vi "createItemsInstances.vi"(8 "error in (no error)":errorcluster, 11 "reference in":refnum<class "Items Controller.lvclass">) -> (0 "error out":errorcluster, 3 "reference out":refnum<class "Items Controller.lvclass">)   [LabVIEW 2016, in "Items Controller.lvclass"]
uses:
  Items Controller.lvclass
  storageSheets.ctl
  APP/item_class/item.lvclass
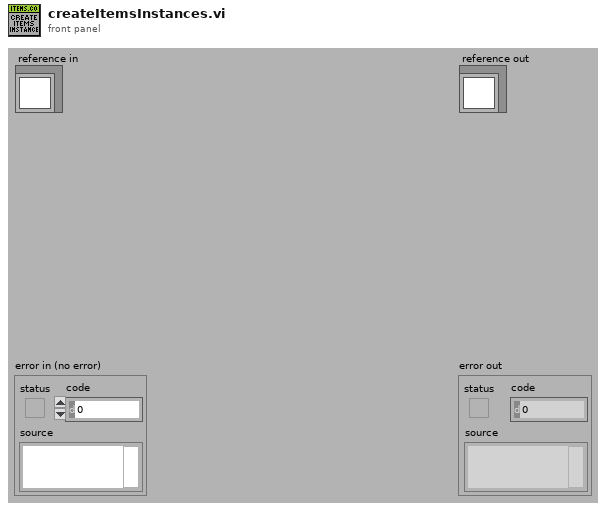
[diagram p1: front panel]
types:
  T1 = typedef "Items Controller.lvclass/storageSheets.ctl" = enum16{"check-in", "check-out", "storage"}
  T2 = typedef "Items Controller.lvclass/ObjectAttributesRef.ctl" = refnum<data-value>
  T3 = typedef "Items Controller.lvclass/ObjectAttributes.ctl" = cluster{"MyAttribute":dbl, "data":string[][][], "file_controller_ref":refnum<class "File Controller.lvclass">, "checkIN_ref":refnum<class "checkIN.lvclass">, "checkOUT_ref":refnum<class "checkOUT.lvclass">, "item_ref":refnum<class "item.lvclass">}
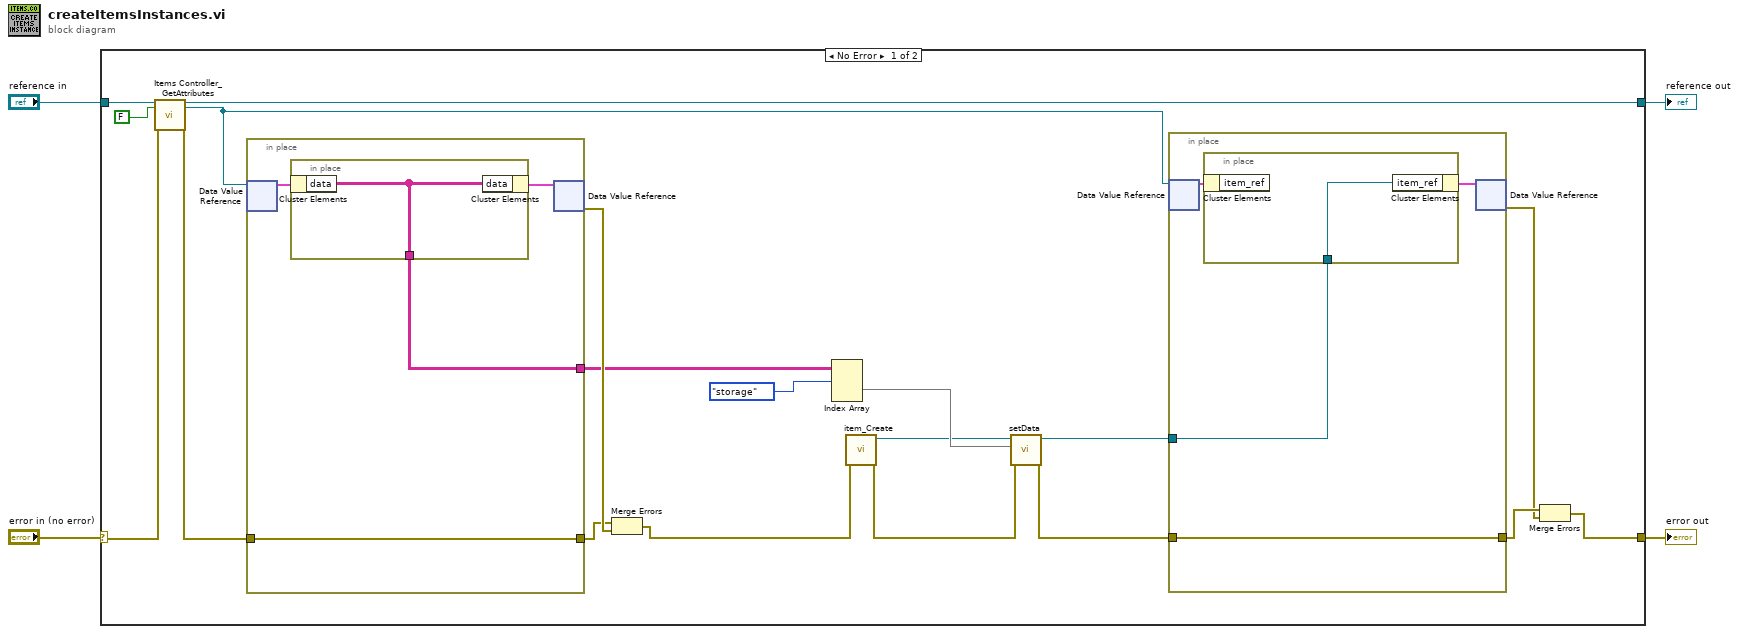
[diagram p0: block diagram]
diagram:
  n1 = case shown="No Error" "error in (no error)" {
    selector: "error in (no error)" -> [w19 w35]
    tunnel: [w12 w35] -> w3
    tunnel: [w17 w34] -> w1
    tunnel: "reference in" -> [w21 w34]
    frame No Error {
      n2 = call "Items Controller_GetAttributes.vi"("reference in"=w21, "return data? (T)"=FALSE, "error in (no error)"=w19) -> ("reference out"=w17:refnum<class "Items Controller.lvclass">, "attributes ref"=w11:T2, "error out"=w18:errorcluster)  [unwired: 13 in, 1 out]
      n3 = in-place {
        in-place-border: w18 -> [w30]
        in-place-border: [w30] -> w22
        in-place-border: [w29] -> w16
        n4 = in-place-dvr #1(w11) -> (w31:T3)  [unwired: 1 out]
        n5 = in-place {
          in-place-border: [w33] -> w29
          n6 = in-place-cluster #2(w31) -> ("data"=w33:string[][][])
          n7 = in-place-cluster #2("data"=w33) -> (w32:T3)
        }
        n8 = in-place-dvr #1(w32) -> (w23:errorcluster)  [unwired: 1 out]
      }
      n9 = Merge Errors(w22, w23) -> (w15:errorcluster)
      n10 = Index Array(array=w16, index (dim 0)=storageSheets."storage" ("storageSheets")) -> (element=w9:string[][])  [unwired: 2 in]
      n11 = call "item_Create.vi"("error in (no error)"=w15) -> ("error out"=w6:errorcluster, "reference out"=w8:refnum<class "item.lvclass">)  [unwired: 9 in]
      n12 = call "setData.vi"("error in (no error)"=w6, "data"=w9, "reference in"=w8) -> ("error out"=w5:errorcluster, "reference out"=w7:refnum<class "item.lvclass">)  [unwired: 7 in]
      n13 = in-place {
        in-place-border: w5 -> [w25]
        in-place-border: [w25] -> w14
        in-place-border: w7 -> [w24]
        n14 = in-place-dvr #3(w11) -> (w26:T3)  [unwired: 1 out]
        n15 = in-place {
          in-place-border: w24 -> [w28]
          n16 = in-place-cluster #4(w26) -> ()  [unwired: 1 out]
          n17 = in-place-cluster #4("item_ref"=w28) -> (w27:T3)
        }
        n18 = in-place-dvr #3(w27) -> (w13:errorcluster)  [unwired: 1 out]
      }
      n19 = Merge Errors(w14, w13) -> (w12:errorcluster)
    }
    frame Error {
    }
  }
  "error out" <- w3
  "reference out" <- w1
